vi "Autonomous Independent.vi"() -> ()   [LabVIEW 2013]
doc: "This VI is called when autonomous begins, and will automatically be terminated when autonomous ends. You can carry out timed or sensor driven robot movement independently without needing to return to the caller."
uses:
  Robot Global Data.vi
panel:
  out "Time":dbl
  out "Hot?":bool
  out "CheckGoalTimedOut?":bool
  in  "CheckHotGoalTimeout":u32=1000
  # "Be sure to right-click and choose Data Operations>>Make Current Value default if you want to save the array values with the VI"
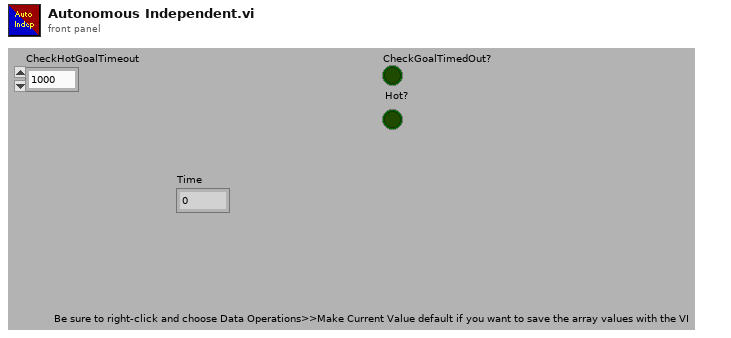
[diagram p1: front panel]
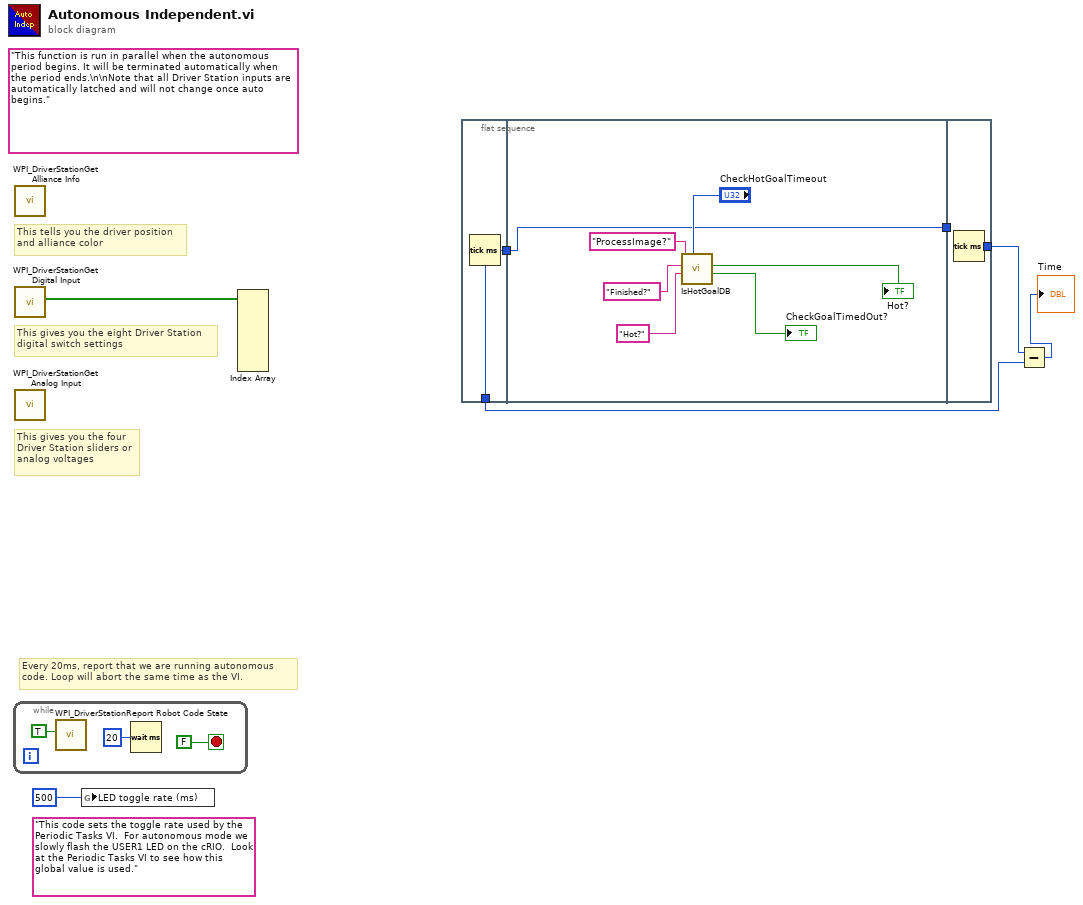
[diagram p0: block diagram]
diagram:
  (unwired) "This code sets the toggle rate used by the Periodic Tasks VI.  For autonomous mode we slowly flash the USER1 LED on the cRIO.  Look at the Periodic Tasks VI to see how this global value is used."
  (unwired) "This function is run in parallel when the autonomous period begins. It will be terminated automatically when the period ends.\n\nNote that all Driver Station inputs are automatically latched and will not change once auto begins."
  # "Every 20ms, report that we are running autonomous\ncode. Loop will abort the same time as the VI."
  # "This tells you the driver position\nand alliance color"
  # "This gives you the eight Driver Station\ndigital switch settings"
  # "This gives you the four\nDriver Station sliders or\nanalog voltages"
  n1 = while {
    stop <- FALSE stop-if-true
    n2 = call <vilib>:"WPI_DriverStationReport Robot Code State.vi"("Autonomous"=TRUE) -> ()  [unwired: 10 in, 1 out]
    n3 = Wait (ms)(milliseconds to wait=u32 20) -> ()  [unwired: 1 out]
  }
  n4 = call <vilib>:"WPI_DriverStationGet Alliance Info.vi"() -> ()  [unwired: 12 out]
  n5 = call <vilib>:"WPI_DriverStationGet Digital Input.vi"() -> ("Driver Station Digital Input (1-8)"=w7:bool[])  [unwired: 11 out]
  n6 = call <vilib>:"WPI_DriverStationGet Analog Input.vi"() -> ()  [unwired: 12 out]
  n7 = global write "Robot Global Data.vi" "LED toggle rate (ms)"(u32 500 ("LED ms toggle rate")) -> ()
  n8 = Index Array(array=w7) -> ()  [unwired: 8 in, 8 out]
  n9 = flat-sequence {
    tunnel: [w11] -> w5
    tunnel: [w11] -> w2
    tunnel: w5 -> [w12]
    tunnel: [w12] -> w4
    tunnel: w4 -> [_]
    tunnel: [w19] -> w3
    frame #0 {
      n10 = Tick Count (ms)() -> (millisecond timer value=w11:u32)
    }
    frame #1 {
      n11 = call "IsHotGoalDB.vi"("Timeout (ms)"="CheckHotGoalTimeout", "DBHot?"="Hot?", "DBFinished?"="Finished?", "DBStart"="ProcessImage?") -> ("TimedOut?"=→"CheckGoalTimedOut?":bool, "Hot?"=→"Hot?":bool)  [unwired: 5 in, 1 out]
    }
    frame #2 {
      n12 = Tick Count (ms)() -> (millisecond timer value=w19:u32)
    }
  }
  n13 = Subtract(x=w3, y=w2) -> (x-y=→"Time":u32)
